vi "Initialise Continuous Capture Mode.vi"(8 "error in":errorcluster, 9 "Data Size":T1, 10 "Buffer Block Size (Samples/Channel)":i32=256, 11 "configuration file path":path) -> (0 "error out":errorcluster)   [LabVIEW 2017, in "DTACQ - Network Enabled Device Driver.lvlib"]
doc: "Prepare the Dtacq device for continuous capture mode"
uses:
  DTACQ - Network Enabled Device Driver.lvlib
  Communications/Typedefs/Data Size--Enum.ctl
  Driver Global Settings--Typedef.ctl
  Communications/Typedefs/DTACQ Connection Data--Cluster.ctl
  FGV Operaions--Enum.ctl
  Communications/Communications Library.lvlib
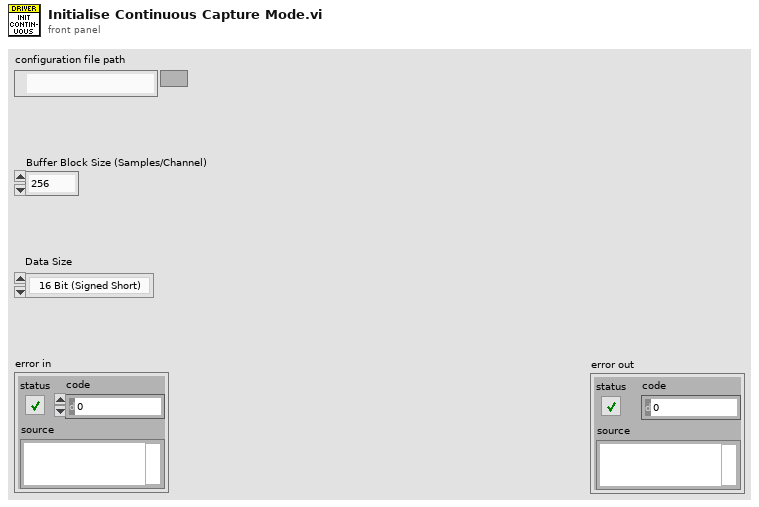
[diagram p1: front panel]
types:
  T1 = typedef "Communications Library.lvlib/Data Size--Enum.ctl" = enum16{"16 Bit (Signed Short)", "32 Bit (Signed Long)"}
  T2 = typedef "DTACQ - Network Enabled Device Driver.lvlib/FGV Operaions--Enum.ctl" = enum16{"Get Driver Settings", "Set Driver Settings", "Search Variable Names", "Close Connections", "Open Connections", "Get Variable References", "Set Variable References", "Clear"}
  T3 = typedef "DTACQ - Network Enabled Device Driver.lvlib/Driver Global Settings--Typedef.ctl" = cluster{"Waveform Length":i32, "Data Size":T1, "DTACQ Connection Data":T4}
  T4 = typedef "Communications Library.lvlib/DTACQ Connection Data--Cluster.ctl" = cluster{"Description":string, "Address":string, "Port":u16, "timeout (ms)":i32, "Termination Character":string, "TCP Connection Reference":refnum<k5>, "Open Connection":bool}
  T5 = typedef "Communications Library.lvlib/DTACQ Module Carrier Configuration--Cluster.ctl" = cluster{"Name":string, "IP":string, "Control Port":i32, "Timeout (ms)":i32, "Continuous Capture Port (Multiplexed)":i32, "Start HIL Shot Port":i32, "AWG Upload Port (Multiplexed)":i32, "Download Captured Data Port (Multiplexed)":i32, "Module Slots":i32, "Module Configurations":T6[]}
  T6 = typedef "Communications Library.lvlib/DTACQ Module Configuration--Cluster.ctl" = cluster{"Name":string, "Position":string, "Module Type":T7, "Control Port":i32, "Timeout (ms)":i32, "Channels":i32}
  T7 = typedef "Communications Library.lvlib/DTACQ Device Type--Enum.ctl" = enum16{"Carrier", "Analog In Module", "Analog Out Module", "Generic Module"}
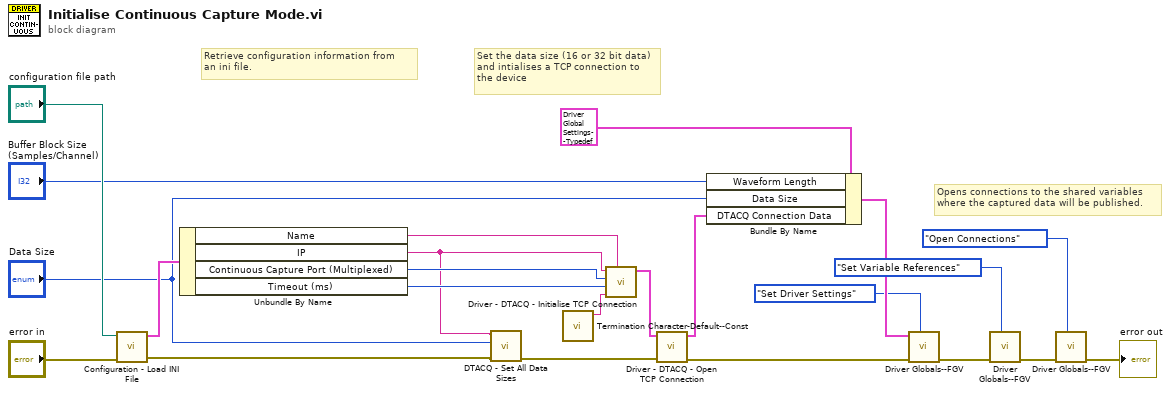
[diagram p0: block diagram]
diagram:
  # "Opens connections to the shared variables\nwhere the captured data will be published."
  # "Set the data size (16 or 32 bit data)\nand intialises a TCP connection to \nthe device"
  # "Retrieve configuration information from\nan ini file."
  n1 = call "Configuration - Load INI File.vi"("error in"="error in", "configuration file path"="configuration file path") -> ("error out"=w4:errorcluster, "Carrier Configuration Out"=w20:T5)  [unwired: 8 in]
  n2 = Unbundle By Name(w20) -> ("Name"=w18:string, "IP"=w2:string, "Continuous Capture Port (Multiplexed)"=w22:i32, "Timeout (ms)"=w21:i32)
  n3 = call "DTACQ - Set All Data Sizes.vi"("error in"=w4, "Analog In Data Size"="Data Size", "Address"=w2) -> ("error out"=w1:errorcluster)  [unwired: 7 in, 1 out]
  n4 = call "Termination Character-Default--Const.vi"() -> ("Termination Character"=w17:string)  [unwired: 11 in]
  n5 = call "Driver - DTACQ - Initialise TCP Connection.vi"("Description"=w18, "Termination Character"=w17, "timeout (ms)"=w21, "Port"=w22, "Address"=w2) -> ("DTACQ Connection Data Out"=w23:T4)  [unwired: 6 in]
  n6 = call "Driver - DTACQ - Open TCP Connection.vi"("error in"=w1, "DTACQ Connection Data In"=w23) -> ("error out"=w10:errorcluster, "DTACQ Connection Data Out"=w13:T4)  [unwired: 8 in]
  n7 = Bundle By Name(cluster=T3 {"Waveform Length"=0, "Data Size"=enum."16 Bit (Signed Short)", "DTACQ Connection Data"={"Description"="", "Address"="", "Port"=0, "timeout (ms)"=5000, "Termination Character"="\n", "TCP Connection Reference"=refnum, "Open Connection"=FALSE}} ("Driver Settings In"), "Waveform Length"="Buffer Block Size (Samples/Channel)", "Data Size"="Data Size", "DTACQ Connection Data"=w13) -> (w12:T3)
  n8 = call "Driver Globals--FGV.vi"(7:FGV_Operaions--Enum."Set Driver Settings", "error in"=w10, "Driver Settings In"=w12) -> ("error out"=w9:errorcluster)  [unwired: 5 in, 3 out]
  n9 = call "Driver Globals--FGV.vi"(7:FGV_Operaions--Enum."Set Variable References", "error in"=w9) -> ("error out"=w8:errorcluster)  [unwired: 6 in, 3 out]
  n10 = call "Driver Globals--FGV.vi"(7:FGV_Operaions--Enum."Open Connections", "error in"=w8) -> ("error out"=→"error out":errorcluster)  [unwired: 6 in, 3 out]
